vi "Multiply.vi"(10 "d":i32, 11 "c":i32) -> (3 "function return":i32)   [LabVIEW 2015, in "SimpleDLLSecond.lvlib"]
doc: "__declspec(dllexport) int Multiply(int c, int d);\n\n__declspec(dllexport) double Multiply(double c, double d);"
uses:
  SimpleDLLSecond.lvlib
  SimpleDLLSecond.dll
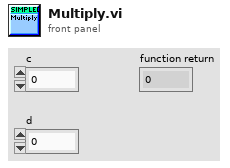
[diagram p1: front panel]
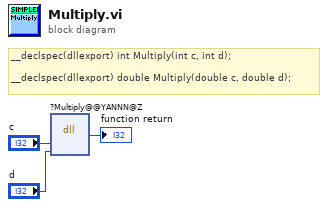
[diagram p0: block diagram]
diagram:
  # "__declspec(dllexport) int Multiply(int c, int d);\n\n__declspec(dllexport) double Multiply(double c, double d);"
  n1 = dll-call lib="C:/Users/adahal/Desktop/AJ/LABVIEW/FirstDLL/SimpleDLLSecond.*" fn="?Multiply@@YANNN@Z"("c"="c", "d"="d") -> (→"function return":i32)  [unwired: 5 in, 2 out]
